vi "Impulse Peak Detector with IC (final value).vi"(2 "init/cont (init:F)":bool, 3 "initial filter state":dbl format="%.2f", 4 "sampling frequency [Hz]":dbl=10000.0 format="%.2f", 5 "X":dbl[](array[numeric]) format="%.2f") -> (0 "final filter state":dbl format="%.2f", 1 "filtered X (final value)":dbl format="%.2f")   [LabVIEW 2017]
doc: "Detects peaks with a decay time constant of 1500 ms on the input signal X and returns only the last value of the filtered signal.\nThe initial filter state and the final filter state parameters keep track of the internal state of the filter to ensure continuous operation of the filter if continuous mode is used."
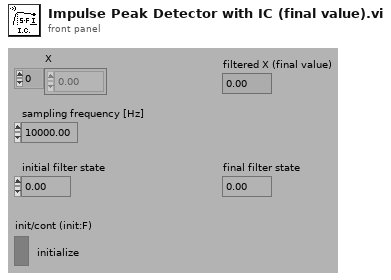
[diagram p1: front panel]
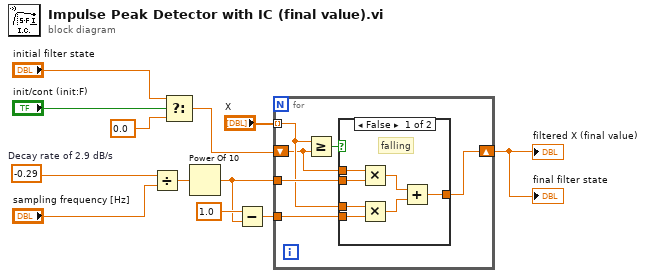
[diagram p0: block diagram]
diagram:
  w12 = -0.29  # Decay rate of 2.9 dB/s
  n1 = Divide(x=w12, y="sampling frequency [Hz]") -> (x/y=w10:dbl)
  n2 = Select(t="initial filter state", s="init/cont (init:F)", f=0.0) -> (s? t:f=w2:dbl)
  n3 = Power Of 10(x=w10) -> (10^x=w7:dbl)
  n4 = Subtract(x=1.0, y=w7) -> (x-y=w6:dbl)
  n5 = for {
    tunnel: "X" -> [w15] mode=indexing
    tunnel: w7 -> [w18]
    tunnel: w6 -> [w17]
    shift-right: [w14] -> w1
    shift-left: w2 -> [w13]
    n6 = Greater Or Equal?(x=w15, y=w13) -> (x >= y?=w16:bool)
    n7 = case shown="False" w16 {
      tunnel: w18 -> [w23 _]
      tunnel: w17 -> [w22 _]
      tunnel: w15 -> [w21 w26]
      tunnel: w13 -> [w20 _]
      tunnel: [w19 w26] -> w14
      frame False {
        # "falling"
        n8 = Multiply(x=w20, y=w23) -> (x*y=w24:dbl)
        n9 = Multiply(x=w21, y=w22) -> (x*y=w25:dbl)
        n10 = Add(x=w24, y=w25) -> (x+y=w19:dbl)
      }
      frame True {
        # "rising"
      }
    }
  }
  "final filter state" <- w1
  "filtered X (final value)" <- w1
